vi "comm timeout.vi"(8 "error in (no error)":errorcluster, 10 "Timeout":u32, 11 "Comm Handle":u64) -> (0 "error out":errorcluster, 3 "dup Comm Handle":u64)   [LabVIEW 2024, in "lvserial.lvlib"]
doc: "Configures the timeout value for read and write operations."
uses:
  <instrlib>/lvserial/lvserial.lvlib
  lvserial.dll
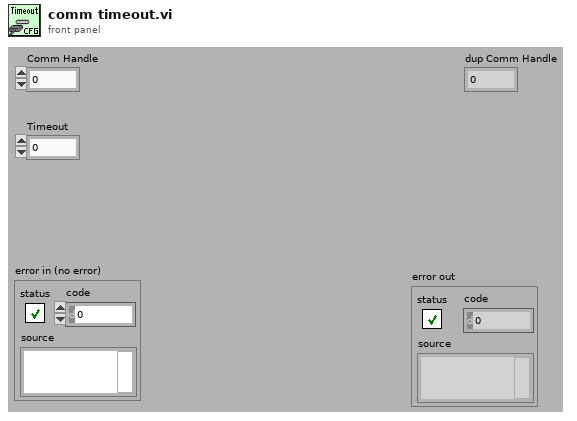
[diagram p1: front panel]
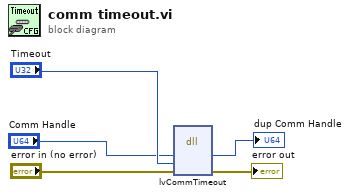
[diagram p0: block diagram]
diagram:
  n1 = dll-call lib="lvserial.dll" fn="lvCommTimeout"("hComm"="Comm Handle", "ulTimeout"="Timeout", "error"="error in (no error)") -> ("hComm"=→"dup Comm Handle":u64, "error"=→"error out":errorcluster)  [unwired: 4 in, 3 out]
